vi "Queue LV2 Driver.vi"(0 "States":string[](array[string]), 2 "Name":string, 11 "Error in":errorcluster, 13 "Operation":T1) -> (4 "Dequeued state":string, 15 "Error out":errorcluster)   [LabVIEW 2020, in "Microwave oven.lvlib"]
doc: "This is a LV2 Queue driven which is used to enqueue and dequeue states in a queue based state machine"
uses:
  Microwave oven.lvlib
  Typedefs/Queue driver operations.ctl
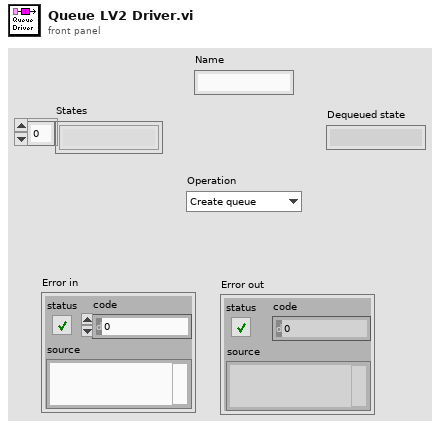
[diagram p1: front panel]
types:
  T1 = typedef "Microwave oven.lvlib/Queue driver operations.ctl" = enum16{"Create queue", "Enqueue", "Enstack", "Dequeue", "Flush", "Release"}
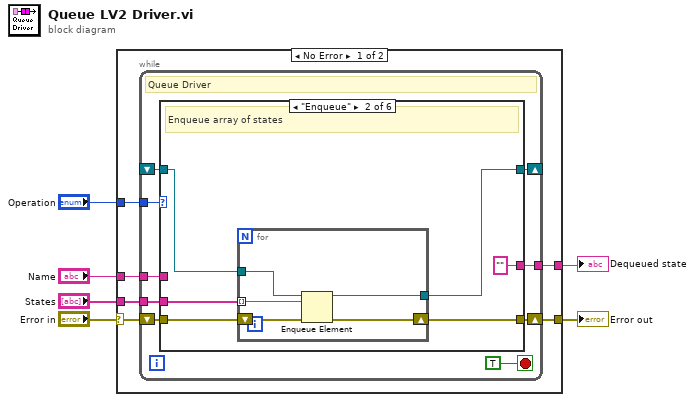
[diagram p0: block diagram]
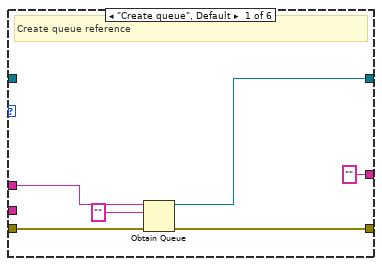
[diagram p2: hidden frame]
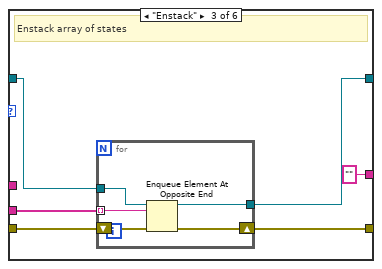
[diagram p3: hidden frame]
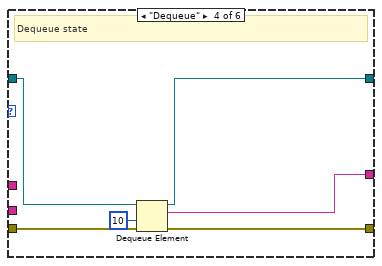
[diagram p4: hidden frame]
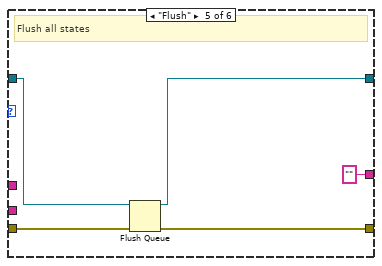
[diagram p5: hidden frame]
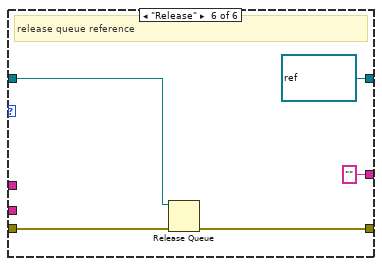
[diagram p6: hidden frame]
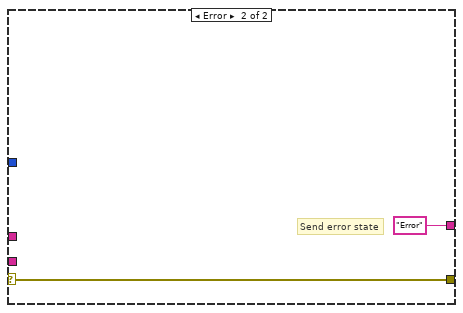
[diagram p7: hidden frame]
diagram:
  n1 = case shown="No Error" "Error in" {
    selector: "Error in" -> [w10 w67]
    tunnel: "Operation" -> [w12 _]
    tunnel: [w11 w67] -> w4
    tunnel: [w9 "Error" ("Dequeued state")] -> w3
    tunnel: "States" -> [w8 _]
    tunnel: "Name" -> [w7 _]
    frame No Error {
      n2 = while {
        tunnel: w12 -> [w21]
        shift-right: [w15] -> _
        shift-left: _ -> [w17]
        shift-right: [w20] -> w11
        shift-left: w10 -> [w19]
        tunnel: [w16] -> w9
        tunnel: w8 -> [w14]
        tunnel: w7 -> [w13]
        stop <- TRUE stop-if-true
        # "Queue Driver"
        n3 = case shown="\"Enqueue\"" w21 {
          tunnel: [w26 w32 w43 w54 w59 w64] -> w20
          tunnel: w19 -> [w27 w33 w44 w55 w60 w65]
          tunnel: w17 -> [_ w31 w42 w52 w58 w63]
          tunnel: ["" "" "" w53 "" ""] -> w16
          tunnel: [w25 w29 w41 w51 w57 refnum<queue> refnum ("queue")] -> w15
          tunnel: w14 -> [_ w30 w40 _ _ _]
          tunnel: w13 -> [w24 _ _ _ _ _]
          frame "Create queue", Default {
            # "Create queue reference"
            n4 = Obtain Queue(name (unnamed)=w24, element data type="" ("Name"), error in (no error)=w27) -> (queue out=w25:refnum<queue>, error out=w26:errorcluster)  [unwired: 2 in, 1 out]
          }
          frame "Enqueue" {
            # "Enqueue array of states"
            n5 = for {
              tunnel: w31 -> [w34]
              tunnel: w30 -> [w36] mode=indexing
              shift-right: [w37] -> w32
              shift-left: w33 -> [w38]
              tunnel: [w35] -> w29
              n6 = Enqueue Element(queue=w34, element=w36, error in (no error)=w38) -> (queue out=w35:refnum<queue>, error out=w37:errorcluster)  [unwired: 1 in, 1 out]
            }
          }
          frame "Enstack" {
            # "Enstack array of states"
            n7 = for {
              tunnel: w42 -> [w47]
              tunnel: [w46] -> w41
              shift-right: [w48] -> w43
              shift-left: w44 -> [w49]
              tunnel: w40 -> [w45] mode=indexing
              n8 = Enqueue Element At Opposite End(queue=w47, element=w45, error in (no error)=w49) -> (queue out=w46:refnum<queue>, error out=w48:errorcluster)  [unwired: 1 in, 1 out]
            }
          }
          frame "Dequeue" {
            # "Dequeue state"
            n9 = Dequeue Element(queue=w52, timeout in ms (-1)=10, error in (no error)=w55) -> (queue out=w51:refnum<queue>, element=w53:string, error out=w54:errorcluster)  [unwired: 1 out]
          }
          frame "Flush" {
            # "Flush all states"
            n10 = Flush Queue(queue=w58, error in (no error)=w60) -> (queue out=w57:refnum<queue>, error out=w59:errorcluster)  [unwired: 1 out]
          }
          frame "Release" {
            # "release queue reference"
            n11 = Release Queue(queue=w63, error in (no error)=w65) -> (error out=w64:errorcluster)  [unwired: 1 in, 2 out]
          }
        }
      }
    }
    frame Error {
      # "Send error state"
    }
  }
  "Dequeued state" <- w3
  "Error out" <- w4
